vi "rotation_mount.vi"(11 "position":dbl) -> (3 "GetPositionCounter":dbl format="%.3f")   [LabVIEW 2016]
uses:
  C:/Users/UsphereLab/Documents/GitHub/Optlev/LabView Code/kinesis/ThorLabs.MotionControl.KCube.DCServoCLI.dll
  kinesis/ThorLabs.MotionControl.KCube.DCServoCLI.dll
  C:/Users/UsphereLab/Documents/GitHub/Optlev/LabView Code/kinesis/Thorlabs.MotionControl.Controls.dll
  kinesis/Thorlabs.MotionControl.Controls.dll
panel:
  in  "acceleration 2":dbl=1.0 format="%#_13g"
  in  "maxVelocity 2":dbl=2.0 format="%#_13g"
  out "acceleration":dbl
  out "maxVelocity":dbl
  in  "stop":bool
  in  "SerialNumber":string="27000959"
  in  "KCubeDCServoControl":refnum<k24>(container)
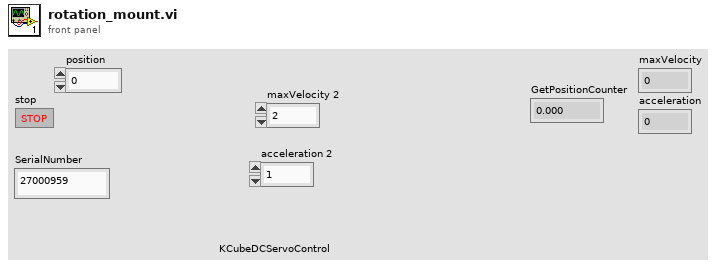
[diagram p1: front panel]
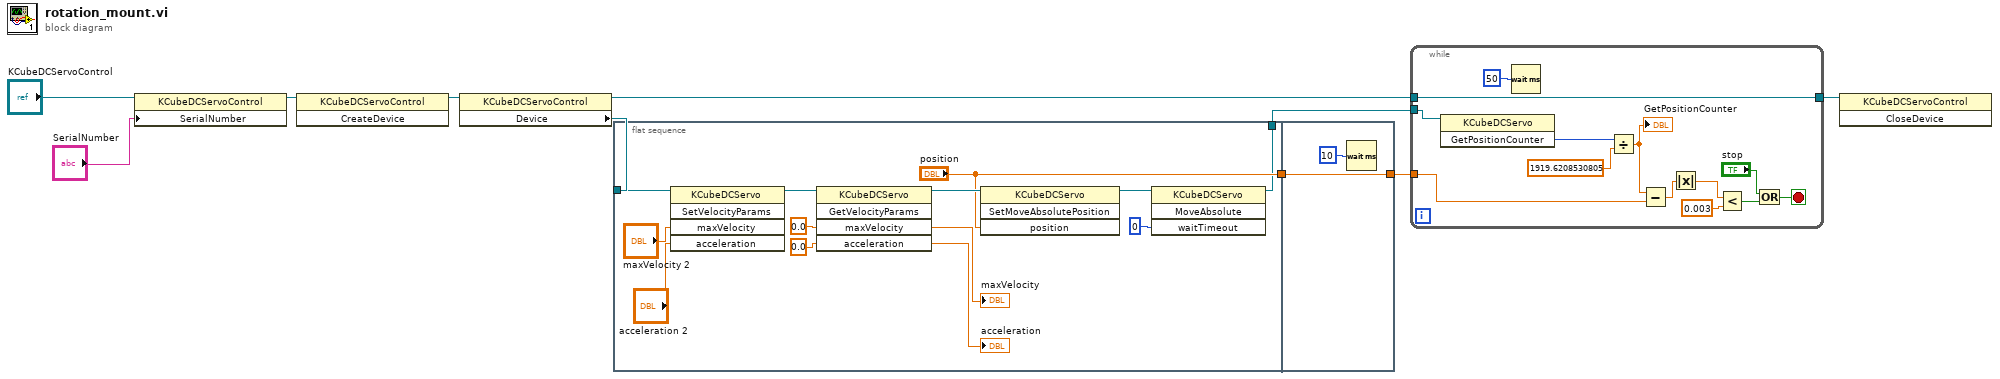
[diagram p0: block diagram]
diagram:
  n1 = property class="KCubeDCServoControl"(reference="KCubeDCServoControl", "SerialNumber"="SerialNumber") -> (reference out=w8:refnum<k24>)  [unwired: 1 in, 1 out]
  n2 = invoke class="KCubeDCServoControl" method="CreateDevice"(reference=w8) -> (reference out=w6:refnum<k24>)  [unwired: 2 in, 2 out]
  n3 = property class="KCubeDCServoControl"(reference=w6) -> (reference out=w5:refnum<k24>, "Device"=w4:refnum<k24>)  [unwired: 1 in, 1 out]
  n4 = flat-sequence {
    tunnel: w4 -> [w16]
    tunnel: ["position"] -> w2
    tunnel: [w11] -> w1
    tunnel: [w25] -> w3
    tunnel: w2 -> [w25]
    frame #0 {
      n5 = invoke class="KCubeDCServo" method="SetVelocityParams"(reference=w16, "maxVelocity"="maxVelocity 2", "acceleration"="acceleration 2") -> (reference out=w15:refnum<k24>)  [unwired: 2 in, 4 out]
      n6 = invoke class="KCubeDCServo" method="GetVelocityParams"(reference=w15, "maxVelocity"=0.0, "acceleration"=0.0) -> (reference out=w21:refnum<k24>, "maxVelocity"=→"maxVelocity":dbl, "acceleration"=→"acceleration":dbl)  [unwired: 2 in, 2 out]
      n7 = invoke class="KCubeDCServo" method="SetMoveAbsolutePosition"(reference=w21, "position"="position") -> (reference out=w22:refnum<k24>)  [unwired: 2 in, 3 out]
      n8 = invoke class="KCubeDCServo" method="MoveAbsolute"(reference=w22, "waitTimeout"=0) -> (reference out=w11:refnum<k24>)  [unwired: 2 in, 3 out]
    }
    frame #1 {
      n9 = Wait (ms)(milliseconds to wait=u32 10) -> ()  [unwired: 1 out]
    }
  }
  n10 = while {
    tunnel: w5 -> [w38]
    tunnel: [w38] -> w7
    tunnel: w3 -> [w32]
    tunnel: w1 -> [w28]
    stop <- w33 stop-if-true
    n11 = invoke class="KCubeDCServo" method="GetPositionCounter"(reference=w28) -> ("GetPositionCounter"=w37:i32)  [unwired: 2 in, 2 out]
    n12 = Wait (ms)(milliseconds to wait=u32 50) -> ()  [unwired: 1 out]
    n13 = Divide(x=w37, y=1919.6208530805) -> (x/y=w31:dbl)
    "GetPositionCounter" <- w31
    n14 = Subtract(x=w31, y=w32) -> (x-y=w27:dbl)
    n15 = Absolute Value(x=w27) -> (abs(x)=w26:dbl)
    n16 = Less?(x=w26, y=0.003) -> (x < y?=w30:bool)
    n17 = Or(x="stop", y=w30) -> (x .or. y?=w33:bool)
  }
  n18 = invoke class="KCubeDCServoControl" method="CloseDevice"(reference=w7) -> ()  [unwired: 2 in, 3 out]
